vi "Max Read Array.vi"(8 "error in":errorcluster, 11 "Max Temperature Limit in":refnum<class "Temperature Limit.lvclass">) -> (0 "error out":errorcluster, 1 "Changed or First Call?":bool, 2 "Temperature Max SP":dbl[](array[numeric]), 3 "Max Temperature Limit out":refnum<class "Temperature Limit.lvclass">)   [LabVIEW 2023, in "Temperature Limit.lvclass"]
uses:
  Temperature Limit.lvclass
  Temperature Limit.lvclass/Temperature Limit.ctl
  Parents/Limit/Limit.lvclass
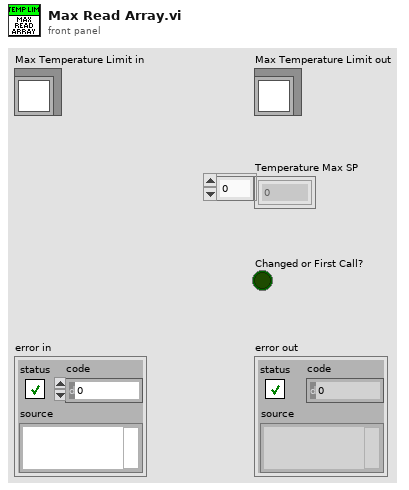
[diagram p1: front panel]
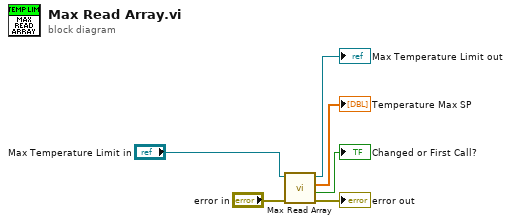
[diagram p0: block diagram]
diagram:
  n1 = call-parent "Max Read Array.vi"("error in"="error in", "Max Limit in"="Max Temperature Limit in") -> ("error out"=→"error out":errorcluster, "Changed or First Call?"=→"Changed or First Call?":bool, "Current Max SP"=→"Temperature Max SP":dbl[], "Max Limit out"=→"Max Temperature Limit out":refnum<class "Temperature Limit.lvclass">)  [unwired: 6 in]
